vi "loop timer.vi"() -> (1 "IPS":dbl, 2 "SPI":u32)   [LabVIEW 2013]
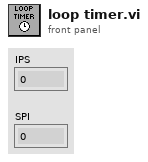
[diagram p1: front panel]
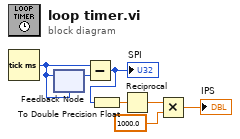
[diagram p0: block diagram]
diagram:
  n1 = Tick Count (ms)() -> (millisecond timer value=w2:u32)
  n2 = feedback #1(w2) -> (w1:u32)
  n3 = feedback-in #1(w2) -> ()
  n4 = Subtract(x=w2, y=w1) -> (x-y=w4:u32)
  "SPI" <- w4
  n5 = To Double Precision Float(number=w4) -> (double precision float=w3:dbl)
  n6 = Reciprocal(x=w3) -> (1/x=w5:dbl)
  n7 = Multiply(x=w5, y=1000.0) -> (x*y=→"IPS":dbl)
